vi "Reverse Heading.vi"(11 "Motion in":refnum<class "Motion.lvclass">) -> (3 "Motion out":refnum<class "Motion.lvclass">)   [LabVIEW 2021, in "Motion.lvclass"]
uses:
  Motion.lvclass
  Motion.lvclass/Motion.ctl
  Math/Math.lvlib
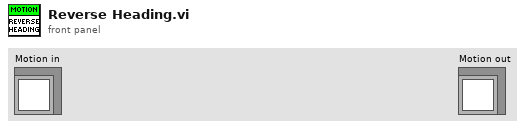
[diagram p1: front panel]
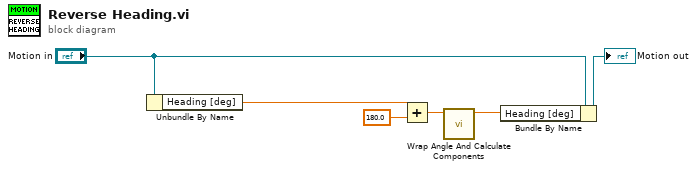
[diagram p0: block diagram]
diagram:
  n1 = Unbundle By Name("Motion in") -> ("Heading [deg]"=w3:sgl)
  n2 = Add(x=w3, y=sgl 180.0) -> (x+y=w2:sgl)
  n3 = call "Wrap Angle And Calculate Components.vi"("Angle in [deg]"=w2) -> ("Angle out [deg]"=w4:sgl)  [unwired: 10 in]
  n4 = Bundle By Name(cluster="Motion in", "Heading [deg]"=w4) -> (→"Motion out":refnum<class "Motion.lvclass">)
